vi "XYStage.DVRtoRef.vi"(10 "Ref":T1) -> (2 "Ref":u32 format="%08x")   [LabVIEW 2015, in "XYStage.lvclass"]
doc: "JKI State Machine Objects (SMO) 1.0.0.5\nJKI - JKI\nCopyright (c) 2016, JKI"
uses:
  XYStage.lvclass
  Typedefs/PrivateData--Ref.ctl
  Typedefs/PrivateData--Cluster.ctl
  Typedefs/Dependencies--Cluster.ctl
  <vilib>/JKI/JKI SMO/SMO.Dictionary.Variant/SMO.Dictionary.Variant.lvclass
  Typedefs/PublicEvents--Cluster.ctl
  Typedefs/(real)Coords--Cluster.ctl
  Typedefs/PublicEvents--XYStage.UpdatedNamedPosition.ctl
  Typedefs/ProtectedEvents--Cluster.ctl
  Typedefs/API Inputs--Cluster.ctl
  Typedefs/PrivateEvents--Cluster.ctl
  Typedefs/PrivateEvents--XYStage.MoveToNamedPosition.ctl
  Typedefs/PrivateEvents--XYStage.StorePosition.ctl
  Typedefs/PrivateEvents--XYStage.Home.ctl
  Typedefs/Configuration--Cluster.ctl
  Typedefs/TargetPositions--Cluster.ctl
  Typedefs/(counts)Coords--Cluster.ctl
  Typedefs/MoveParameters--Cluster.ctl
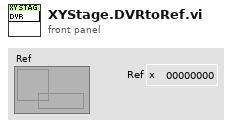
[diagram p1: front panel]
types:
  T1 = typedef "XYStage.lvclass/PrivateData--Ref.ctl" = refnum<data-value>
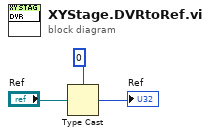
[diagram p0: block diagram]
diagram:
  n1 = Type Cast(type=u32 0 ("Ref"), x="Ref") -> (*(type *) &x=→"Ref":u32)
